vi "encodeStream.vi"(8 "error in (no error)":errorcluster, 11 "tBSONNull in":refnum<class "tBSONNull.lvclass">) -> (0 "error out":errorcluster, 2 "Byte Array":u8[](array[numeric]), 3 "tBSONNull out":refnum<class "tBSONNull.lvclass">)   [LabVIEW 2013, in "BSON.lvlib" / "tBSONNull.lvclass"]
uses:
  tBSONNull.lvclass
  tBSONElement/tBSONElement.lvclass
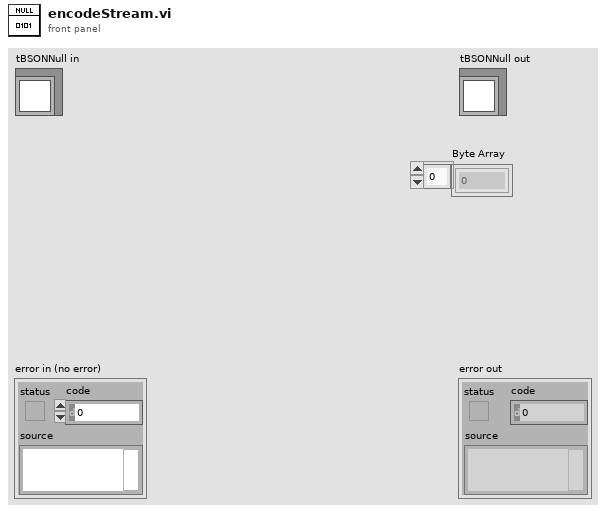
[diagram p1: front panel]
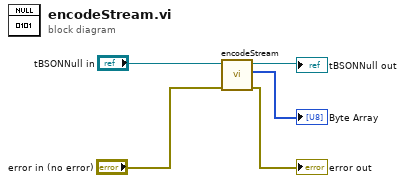
[diagram p0: block diagram]
diagram:
  n1 = call-parent "encodeStream.vi"("error in (no error)"="error in (no error)", "tBSONElement in"="tBSONNull in") -> ("error out"=→"error out":errorcluster, "Byte Array"=→"Byte Array":u8[], "tBSONElement out"=→"tBSONNull out":refnum<class "tBSONNull.lvclass">)  [unwired: 7 in]
